vi "destKickFactorPass.vi"(6 "dest_y_kick":dbl, 9 "dest_x_kick":dbl, 10 "Game in":refnum<class "Game.lvclass">, 11 "Utilities in":refnum<class "Utilities.lvclass">) -> (2 "FactorPass":dbl[](array[numeric]), 3 "Debug":dbl[][](array[numeric]))   [LabVIEW 2020, in "5RobotsPassGamePlay.lvclass"]
uses:
  5RobotsPassGamePlay.lvclass
  Game_class/Game.lvclass
  Utilities_class/Utilities.lvclass
  Game_class/Game.lvclass/Game.ctl
  Game_class/Read FieldRef.vi
  Field_class/Field.lvclass
  5RobotsPassGamePlay.lvclass/5RobotsPassGamePlay.ctl
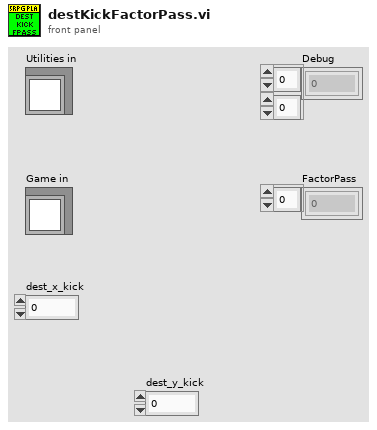
[diagram p1: front panel]
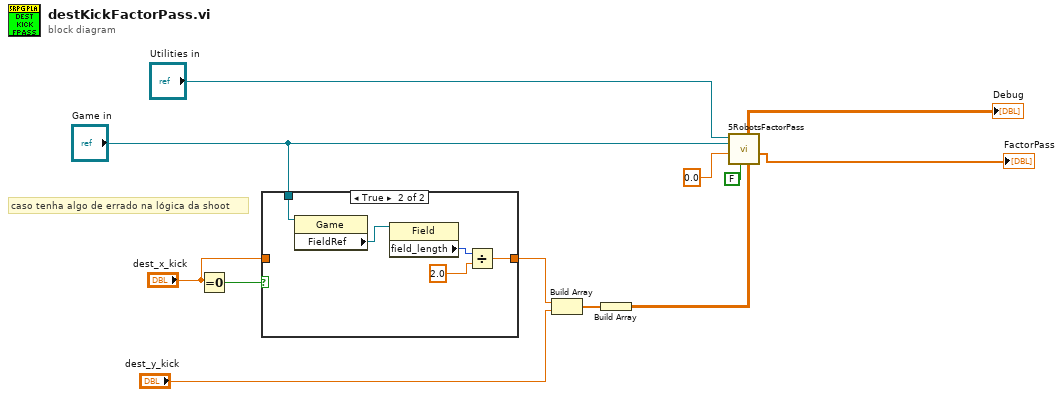
[diagram p0: block diagram]
diagram:
  # "caso tenha algo de errado na lógica da shoot"
  n1 = Equal To 0?(x="dest_x_kick") -> (x = 0?=w4:bool)
  n2 = case shown="True" w4 {
    tunnel: "Game in" -> [_ w16]
    tunnel: [w13 w14] -> w2
    tunnel: "dest_x_kick" -> [w13 _]
    frame False {
    }
    frame True {
      n3 = property class="Game"(reference=w16) -> ("FieldRef"=w15:refnum<class "Field.lvclass">)  [unwired: 1 in, 2 out]
      n4 = property class="Field"(reference=w15) -> ("field_length"=w18:i32)  [unwired: 1 in, 2 out]
      n5 = Divide(x=w18, y=2.0) -> (x/y=w14:dbl)
    }
  }
  n6 = Build Array(w2, "dest_y_kick") -> (w6:dbl[])
  n7 = Build Array(w6) -> (w5:dbl[][])
  n8 = call-dynamic "5RobotsFactorPass.vi"("dest_kick"=w5, "Pass?"=FALSE, "Root"=0.0, "Game in"="Game in", "Utilities in"="Utilities in") -> ("FactorPass"=→"FactorPass":dbl[], "Debug"=→"Debug":dbl[][])  [unwired: 2 in, 3 out]
